vi "Read from File.vi"(8 "error in (no error)":errorcluster, 11 "file path":path) -> (0 "error out":errorcluster, 2 "digital audio protocol settings":T1, 5 "file exists?":bool)   [LabVIEW 2021, in "digital audio protocol controls.lvlib"]
uses:
  digital audio protocol controls.lvlib
  digital audio protocol settings.ctl
  digital audio protocol settings_json.ctl
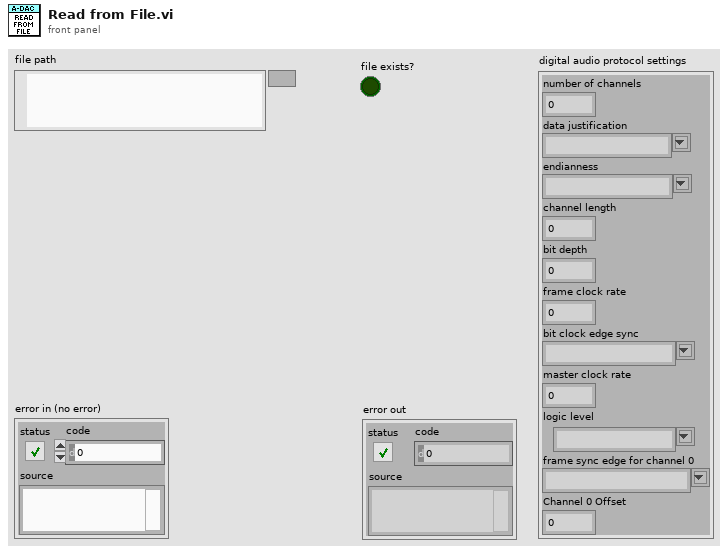
[diagram p1: front panel]
types:
  T1 = typedef "digital audio protocol controls.lvlib/digital audio protocol settings.ctl" = cluster{"number of channels":u32, "data justification":string, "endianness":string, "channel length":u32, "bit depth":u32, "frame clock rate":dbl, "bit clock edge sync":string, "master clock rate":dbl, "logic level":string, "frame sync edge for channel 0":string, "Channel 0 Offset":u32}
  T2 = typedef "digital audio protocol controls.lvlib/digital audio protocol settings_json.ctl" = cluster{"number of channels":u32, "data justification":string, "endianness":string, "channel length":u32, "bit depth":u32, "frame clock rate":dbl, "bit clock edge sync":string, "master clock rate":dbl, "logic level":string, "frame sync edge for channel 0":string, "Channel 0 Offset":u32}
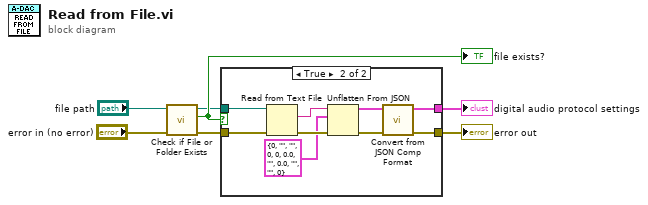
[diagram p0: block diagram]
diagram:
  n1 = call <vilib>:"Check if File or Folder Exists.vi"("error in (no error)"="error in (no error)", "path"="file path") -> ("error out"=w6:errorcluster, "file or folder exists?"=w5:bool, "dup path"=w4:path)  [unwired: 7 in]
  "file exists?" <- w5
  n2 = case shown="True" w5 {
    tunnel: w6 -> [w8 w16]
    tunnel: w4 -> [_ w17]
    tunnel: [_ w11] -> w1
    tunnel: [w8 w9] -> w2
    frame False {
      # "no file found"
    }
    frame True {
      n3 = Read from Text File(file (use dialog)=w17, error in=w16) -> (text=w14:string, error out=w15:errorcluster)  [unwired: 2 in, 2 out]
      n4 = Unflatten From JSON(JSON string=w14, type and defaults=T2 {"number of channels"=0, "data justification"="", "endianness"="", "channel length"=0, "bit depth"=0, "frame clock rate"=0.0, "bit clock edge sync"="", "master clock rate"=0.0, "logic level"="", "frame sync edge for channel 0"="", "Channel 0 Offset"=0} ("digital audio protocol settings"), error in (no error)=w15) -> (value=w12:T2, error out=w10:errorcluster)  [unwired: 4 in]
      n5 = call "Convert from JSON Comp Format.vi"("error in (no error)"=w10, "JSON format"=w12) -> ("error out"=w9:errorcluster, "digital audio protocol settings"=w11:T1)  [unwired: 8 in]
    }
  }
  "digital audio protocol settings" <- w1
  "error out" <- w2
